vi "TxBfrPkt - Init Packet Page.vi"(6 "Tx Buffered Data Packet Refs":T1, 8 "error in (no error)":errorcluster, 11 "Node Ptr In":T2 format="%.0x") -> (0 "error out":errorcluster, 3 "Node Ptr Out":T2 format="%.0x")   [LabVIEW 2016, in "UDP-Custom-Device System Explorer.lvlib"]
uses:
  UDP-Custom-Device System Explorer.lvlib
  <vilib>/NI Veristand/Custom Device API/Custom Device Item Ref.ctl
  Types/Page References/Refs - Tx Buffered Data Packet Page.ctl
  Shared/Types/Shared - Transmit Buffer Options.ctl
  Shared/Types/Shared - Transmit Sim Options.ctl
  <vilib>/NI VeriStand/Custom Device API/Custom Device API.lvlib
  Property Accessors/Shared Packet Accessors.lvlib
  Property Accessors/Buffered Data Packet.lvlib
  Property Accessors/Tx Packet Accessors.lvlib
  Shared/UDP-Custom-Device Shared.lvlib
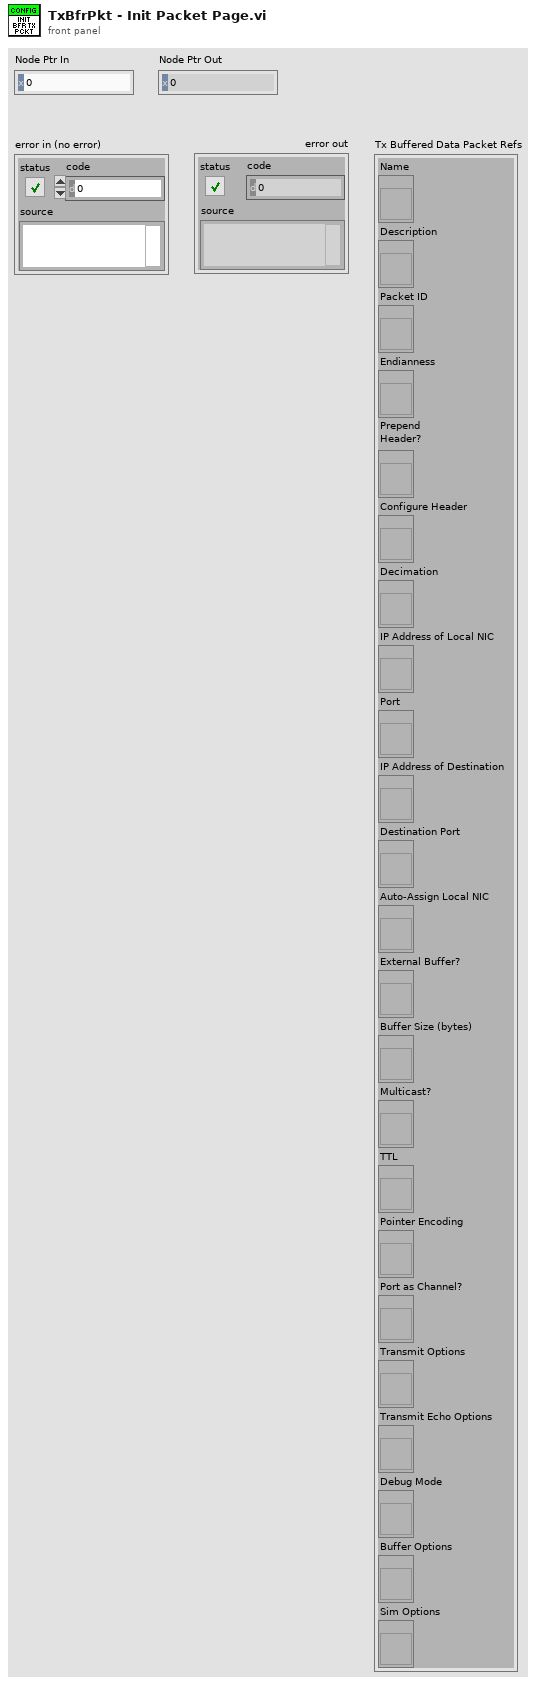
[diagram p1: front panel]
types:
  T1 = typedef "UDP-Custom-Device System Explorer.lvlib/Refs - Tx Buffered Data Packet Page.ctl" = cluster{"Name":refnum<vi>, "Description":refnum<vi>, "Packet ID":refnum<vi>, "Endianness":refnum<vi>, "Prepend\nHeader?":refnum<vi>, "Configure Header":refnum<vi>, "Decimation":refnum<vi>, "IP Address of Local NIC":refnum<vi>, "Port":refnum<vi>, "IP Address of Destination":refnum<vi>, "Destination Port":refnum<vi>, "Auto-Assign Local NIC":refnum<vi>, "External Buffer?":refnum<vi>, "Buffer Size (bytes)":refnum<vi>, "Multicast?":refnum<vi>, "TTL":refnum<vi>, "Pointer Encoding":refnum<vi>, "Port as Channel?":refnum<vi>, "Transmit Options":refnum<vi>, "Transmit Echo Options":refnum<vi>, "Debug Mode":refnum<vi>, "Buffer Options":refnum<vi>, "Sim Options":refnum<vi>}
  T2 = typedef "Custom Device API.lvlib/Custom Device Item Ref.ctl" = u64
  T3 = typedef "UDP-Custom-Device Shared.lvlib/Shared - Transmit Sim Options.ctl" = enum16{"No Simulation", "Counter", "Full Buffer", "FIFO Test", "FIFO + Port Test"}
  T4 = typedef "UDP-Custom-Device Shared.lvlib/Shared - Transmit Buffer Options.ctl" = enum16{"Static Buffer", "FIFO Buffer", "FIFO Buffer + Port"}
  T5 = enum8{"Enabled", "Disabled", "Disabled and Grayed Out"}
  T6 = typedef "UDP-Custom-Device Shared.lvlib/Shared - Transmit Echo Options.ctl" = enum16{"PCL Reset", "Counter", "Mirror"}
  T7 = typedef "UDP-Custom-Device Shared.lvlib/Shared - Pointer Encoding.ctl" = enum16{"Direct Encoding", "Conversion Encoding"}
  T8 = typedef "UDP-Custom-Device Shared.lvlib/Shared - Transmit Flag Options.ctl" = enum16{"Always", "One-Shot", "Toggle"}
  T9 = typedef "Custom Device API.lvlib/Custom Device Item Info.ctl" = cluster{"Name":string, "Is Channel":bool, "GUID":string, "Is Waveform":bool}
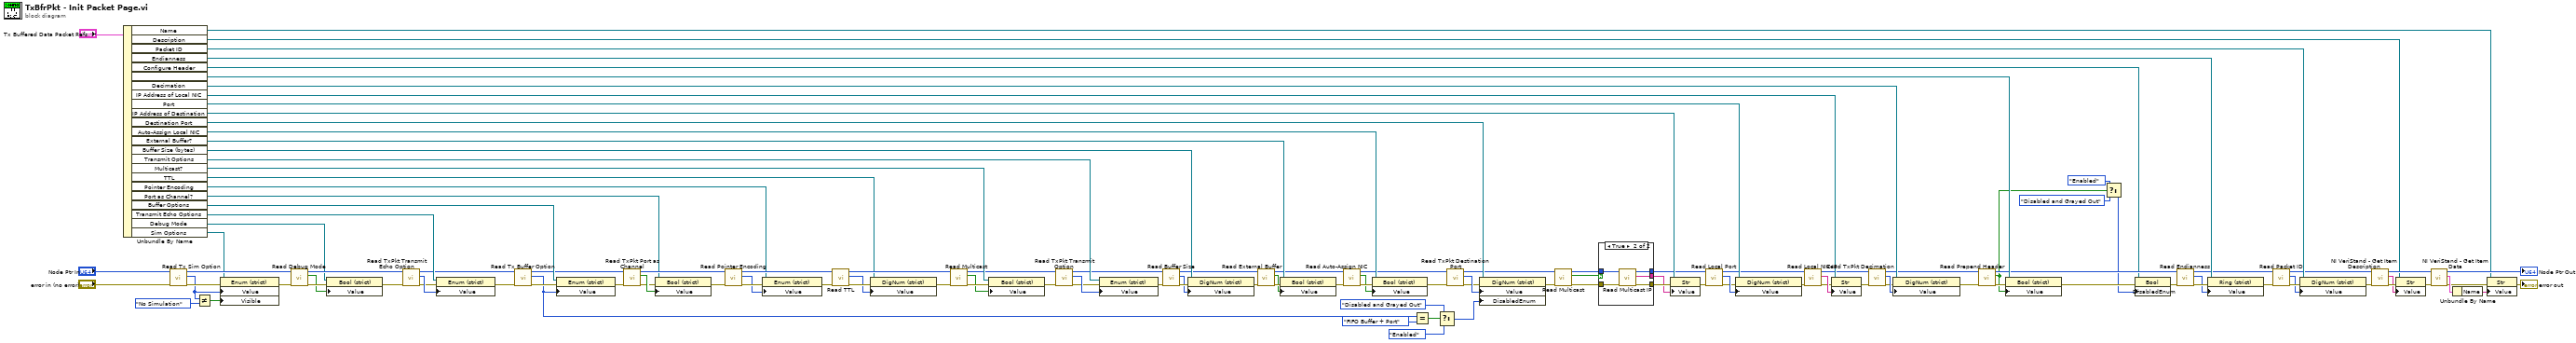
[diagram p0: block diagram]
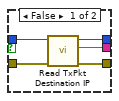
[diagram p2: hidden frame]
diagram:
  n1 = Unbundle By Name("Tx Buffered Data Packet Refs") -> ("Name"=w119:refnum<vi>, "Description"=w118:refnum<vi>, "Packet ID"=w117:refnum<vi>, "Endianness"=w110:refnum<vi>, "Configure Header"=w99:refnum<vi>, "Prepend\nHeader?"=w107:refnum<vi>, "Decimation"=w97:refnum<vi>, "IP Address of Local NIC"=w92:refnum<vi>, "Port"=w86:refnum<vi>, "IP Address of Destination"=w80:refnum<vi>, "Destination Port"=w77:refnum<vi>, "Auto-Assign Local NIC"=w73:refnum<vi>, "External Buffer?"=w69:refnum<vi>, "Buffer Size (bytes)"=w67:refnum<vi>, "Transmit Options"=w59:refnum<vi>, "Multicast?"=w53:refnum<vi>, "TTL"=w51:refnum<vi>, "Pointer Encoding"=w43:refnum<vi>, "Port as Channel?"=w38:refnum<vi>, "Buffer Options"=w29:refnum<vi>, "Transmit Echo Options"=w27:refnum<vi>, "Debug Mode"=w23:refnum<vi>, "Sim Options"=w6:refnum<vi>)
  n2 = call "Read Tx Sim Option.vi"("error in (no error)"="error in (no error)", "Node Ptr"="Node Ptr In") -> ("error out"=w5:errorcluster, "Sim Option"=w3:T3, "Node Ptr out"=w8:T2)  [unwired: 7 in]
  n3 = Not Equal?(x=w3, y=Shared_-_Transmit_Sim_Options."No Simulation") -> (x != y?=w1:bool)
  n4 = property class="Enum (strict)"(reference=w6, error in=w5, "Value"=w3, "Visible"=w1) -> (error out=w4:errorcluster)  [unwired: 1 out]
  n5 = call "Read Debug Mode.vi"("error in (no error)"=w4, "Node Ptr"=w8) -> ("error out"=w22:errorcluster, "Debug Mode"=w20:bool, "Node Ptr out"=w25:T2)  [unwired: 7 in]
  n6 = property class="Bool (strict)"(reference=w23, error in=w22, "Value"=w20) -> (error out=w21:errorcluster)  [unwired: 1 out]
  n7 = call "Read TxPkt Transmit Echo Option.vi"("error in (no error)"=w21, "Node Ptr"=w25) -> ("error out"=w24:errorcluster, "Transmit Echo Options"=w26:T6, "Node Ptr out"=w19:T2)  [unwired: 7 in]
  n8 = property class="Enum (strict)"(reference=w27, error in=w24, "Value"=w26) -> (error out=w18:errorcluster)  [unwired: 1 out]
  n9 = call "Read Tx Buffer Option.vi"("error in (no error)"=w18, "Node Ptr"=w19) -> ("error out"=w17:errorcluster, "Buffer Option"=w12:T4, "Node Ptr out"=w16:T2)  [unwired: 7 in]
  n10 = property class="Enum (strict)"(reference=w29, error in=w17, "Value"=w12) -> (error out=w28:errorcluster)  [unwired: 1 out]
  n11 = call "Read TxPkt Port as Channel.vi"("error in (no error)"=w28, "Node Ptr"=w16) -> ("error out"=w36:errorcluster, "Port as Channel"=w37:bool, "Node Ptr out"=w39:T2)  [unwired: 7 in]
  n12 = property class="Bool (strict)"(reference=w38, error in=w36, "Value"=w37) -> (error out=w35:errorcluster)  [unwired: 1 out]
  n13 = call "Read Pointer Encoding.vi"("error in (no error)"=w35, "Node Ptr"=w39) -> ("error out"=w41:errorcluster, "Pointer Encoding"=w40:T7, "Node Ptr out"=w44:T2)  [unwired: 7 in]
  n14 = property class="Enum (strict)"(reference=w43, error in=w41, "Value"=w40) -> (error out=w42:errorcluster)  [unwired: 1 out]
  n15 = call "Read TTL.vi"("error in (no error)"=w42, "Node Ptr"=w44) -> ("error out"=w55:errorcluster, "TTL"=w50:u16, "Node Ptr out"=w57:T2)  [unwired: 7 in]
  n16 = property class="DigNum (strict)"(reference=w51, error in=w55, "Value"=w50) -> (error out=w56:errorcluster)  [unwired: 1 out]
  n17 = call "Read Multicast.vi"("error in (no error)"=w56, "Node Ptr"=w57) -> ("error out"=w54:errorcluster, "Multicast"=w52:bool, "Node Ptr out"=w34:T2)  [unwired: 7 in]
  n18 = property class="Bool (strict)"(reference=w53, error in=w54, "Value"=w52) -> (error out=w33:errorcluster)  [unwired: 1 out]
  n19 = call "Read TxPkt Transmit Option.vi"("error in (no error)"=w33, "Node Ptr"=w34) -> ("error out"=w31:errorcluster, "Transmit Options"=w32:T8, "Node Ptr out"=w30:T2)  [unwired: 7 in]
  n20 = property class="Enum (strict)"(reference=w59, error in=w31, "Value"=w32) -> (error out=w58:errorcluster)  [unwired: 1 out]
  n21 = call "Read Buffer Size.vi"("error in (no error)"=w58, "Node Ptr"=w30) -> ("error out"=w61:errorcluster, "Buffer Size"=w60:u32, "Node Ptr out"=w66:T2)  [unwired: 7 in]
  n22 = property class="DigNum (strict)"(reference=w67, error in=w61, "Value"=w60) -> (error out=w64:errorcluster)  [unwired: 1 out]
  n23 = call "Read External Buffer.vi"("error in (no error)"=w64, "Node Ptr"=w66) -> ("error out"=w63:errorcluster, "External Buffer"=w62:bool, "Node Ptr out"=w65:T2)  [unwired: 7 in]
  n24 = property class="Bool (strict)"(reference=w69, error in=w63, "Value"=w62) -> (error out=w68:errorcluster)  [unwired: 1 out]
  n25 = call "Read Auto-Assign NIC.vi"("error in (no error)"=w68, "Node Ptr"=w65) -> ("error out"=w72:errorcluster, "Auto-Assign NIC"=w71:bool, "Node Ptr out"=w70:T2)  [unwired: 7 in]
  n26 = property class="Bool (strict)"(reference=w73, error in=w72, "Value"=w71) -> (error out=w74:errorcluster)  [unwired: 1 out]
  n27 = Equal?(x=w12, y=Shared_-_Transmit_Buffer_Options."FIFO Buffer + Port") -> (x = y?=w10:bool)
  n28 = Select(t=T5."Disabled and Grayed Out" ("Disabled"), s=w10, f=T5."Enabled" ("Disabled")) -> (s? t:f=w13:T5)
  n29 = call "Read TxPkt Destination Port.vi"("error in (no error)"=w74, "Node Ptr"=w70) -> ("error out"=w75:errorcluster, "Destination Port"=w76:u16, "Node Ptr out"=w49:T2)  [unwired: 7 in]
  n30 = property class="DigNum (strict)"(reference=w77, error in=w75, "Value"=w76, "DisabledEnum"=w13) -> (error out=w47:errorcluster)  [unwired: 1 out]
  n31 = call "Read Multicast.vi"("error in (no error)"=w47, "Node Ptr"=w49) -> ("error out"=w46:errorcluster, "Multicast"=w45:bool, "Node Ptr out"=w48:T2)  [unwired: 7 in]
  n32 = case shown="True" w45 {
    tunnel: [w134 w135] -> w81
    tunnel: [w133 w136] -> w79
    tunnel: [w132 w137] -> w78
    tunnel: w48 -> [w131 w139]
    tunnel: w46 -> [w130 w138]
    frame False {
      n33 = call "Read TxPkt Destination IP.vi"("error in (no error)"=w130, "Node Ptr"=w131) -> ("error out"=w134:errorcluster, "Destination IP"=w133:string, "Node Ptr out"=w132:T2)  [unwired: 7 in]
    }
    frame True {
      n34 = call "Read Multicast IP.vi"("error in (no error)"=w138, "Node Ptr"=w139) -> ("error out"=w135:errorcluster, "Multicast IP Address"=w136:string, "Node Ptr out"=w137:T2)  [unwired: 7 in]
    }
  }
  n35 = property class="Str"(reference=w80, error in=w81, "Value"=w79) -> (error out=w82:errorcluster)  [unwired: 1 out]
  n36 = call "Read Local Port.vi"("error in (no error)"=w82, "Node Ptr"=w78) -> ("error out"=w84:errorcluster, "Port"=w85:u16, "Node Ptr out"=w83:T2)  [unwired: 7 in]
  n37 = property class="DigNum (strict)"(reference=w86, error in=w84, "Value"=w85) -> (error out=w87:errorcluster)  [unwired: 1 out]
  n38 = call "Read Local NIC IP.vi"("error in (no error)"=w87, "Node Ptr"=w83) -> ("error out"=w89:errorcluster, "IP Address of Local NIC"=w90:string, "Node Ptr out"=w88:T2)  [unwired: 7 in]
  n39 = property class="Str"(reference=w92, error in=w89, "Value"=w90) -> (error out=w91:errorcluster)  [unwired: 1 out]
  n40 = call "Read TxPkt Decimation.vi"("error in (no error)"=w91, "Node Ptr"=w88) -> ("error out"=w95:errorcluster, "Decimation"=w96:u16, "Node Ptr out"=w93:T2)  [unwired: 7 in]
  n41 = property class="DigNum (strict)"(reference=w97, error in=w95, "Value"=w96) -> (error out=w94:errorcluster)  [unwired: 1 out]
  n42 = call "Read Prepend Header.vi"("error in (no error)"=w94, "Node Ptr"=w93) -> ("error out"=w106:errorcluster, "Prepend Header"=w102:bool, "Node Ptr out"=w105:T2)  [unwired: 7 in]
  n43 = property class="Bool (strict)"(reference=w107, error in=w106, "Value"=w102) -> (error out=w101:errorcluster)  [unwired: 1 out]
  n44 = Select(t=T5."Enabled" ("Disabled"), s=w102, f=T5."Disabled and Grayed Out" ("Disabled")) -> (s? t:f=w98:T5)
  n45 = property class="Bool"(reference=w99, error in=w101, "DisabledEnum"=w98) -> (error out=w100:errorcluster)  [unwired: 1 out]
  n46 = call "Read Endianness.vi"("error in (no error)"=w100, "Node Ptr"=w105) -> ("error out"=w111:errorcluster, "Endianness"=w109:u16, "Node Ptr out"=w108:T2)  [unwired: 7 in]
  n47 = property class="Ring (strict)"(reference=w110, error in=w111, "Value"=w109) -> (error out=w112:errorcluster)  [unwired: 1 out]
  n48 = call "Read Packet ID.vi"("error in (no error)"=w112, "Node Ptr"=w108) -> ("error out"=w114:errorcluster, "Packet ID"=w113:i32, "Node Ptr out"=w115:T2)  [unwired: 7 in]
  n49 = property class="DigNum (strict)"(reference=w117, error in=w114, "Value"=w113) -> (error out=w116:errorcluster)  [unwired: 1 out]
  n50 = call <vilib>:"NI VeriStand - Get Item Description.vi"("error in (no error)"=w116, "Item Ref in"=w115) -> ("error out"=w126:errorcluster, "Description"=w125:string, "Item Ref out"=w123:T2)  [unwired: 7 out]
  n51 = property class="Str"(reference=w118, error in=w126, "Value"=w125) -> (error out=w124:errorcluster)  [unwired: 1 out]
  n52 = call <vilib>:"NI VeriStand - Get Item Data.vi"("error in (no error)"=w124, "Item Ref in"=w123) -> ("error out"=w127:errorcluster, "Item Info"=w128:T9, "Item Ref out"=→"Node Ptr Out":T2)  [unwired: 6 in, 1 out]
  n53 = Unbundle By Name(w128) -> ("Name"=w122:string)
  n54 = property class="Str"(reference=w119, error in=w127, "Value"=w122) -> (error out=→"error out":errorcluster)  [unwired: 1 out]
